vi "FdxCmdMonQueueStatusCvi.vi"(8 "error in":errorcluster, 10 "QueueId":u32, 11 "InstrumentHandle_port":u32) -> (0 "error out":errorcluster, 1 "QueueStatus":T1 {"QueueStatus" items=["FDX_MON_STAT_EMPTY", "FDX_MON_STAT_ FILLED", "FDX_MON_STAT_ FULL", "FDX_MON_STAT_ OVERFLOW", "FDX_MON_STAT_ ERROR"]}, 3 "InstrumentHandle_port":u32)   [LabVIEW 2020, in "AIM664LV.lvlib"]
uses:
  AIM664LV.lvlib
  AFDX_LibraryAdmin/FdxGlobalDllPath.vi
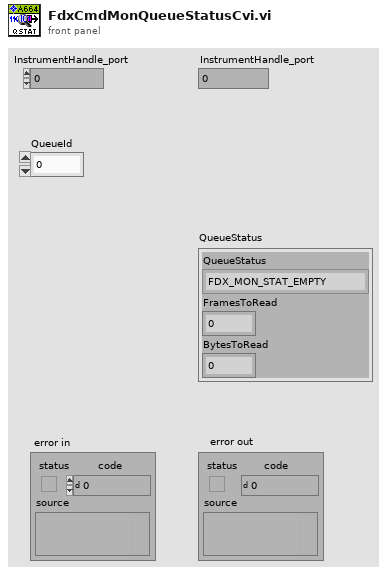
[diagram p1: front panel]
types:
  T1 = cluster{"QueueStatus":u32, "FramesToRead":u32, "BytesToRead":u32}
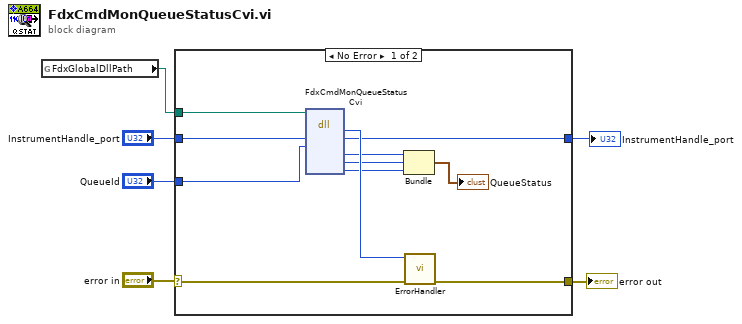
[diagram p0: block diagram]
diagram:
  n1 = global read "FdxGlobalDllPath.vi" "FdxGlobalDllPath"() -> (w4:path)
  n2 = case shown="No Error" "error in" {
    selector: "error in" -> [w16 w19]
    tunnel: [w17 w19] -> w6
    tunnel: w4 -> [w11 _]
    tunnel: "InstrumentHandle_port" -> [w9 w18]
    tunnel: [w8 w18] -> w2
    tunnel: "QueueId" -> [w7 _]
    frame No Error {
      n3 = dll-call lib="aim_fdx.19.dll" fn="FdxCmdMonQueueStatusCvi"(path in=w11, "InstrumentHandle"=w9, "QueueId"=w7) -> ("status"=w15:i32, "InstrumentHandle"=w8:u32, "QueueStatus"=w12:u32, "FramesToRead"=w13:u32, "BytesToRead"=w14:u32)  [unwired: 6 in, 2 out]
      n4 = Bundle("QueueStatus"=w12, "FramesToRead"=w13, "BytesToRead"=w14) -> (→"QueueStatus":T1)  [unwired: 1 in]
      n5 = call "ErrorHandler.vi"("error in"=w16, "AIM Error"=w15) -> ("error out"=w17:errorcluster)  [unwired: 9 in]
    }
    frame Error {
    }
  }
  "error out" <- w6
  "InstrumentHandle_port" <- w2
